vi "SEQ Header Save.vi"(0 "refnum":refnum<file>, 1 "time of 1st frame, \nsec since 1/1/04":dbl format="%.2f", 5 "User Info":string="123456789012345678901234567890123456789", 7 "Description":string="1234567890123456789012345678901234567890123456789012345678901234567890123456789012345678901234567890123456789012345678901234567", 9 "# of Frames":u32=1, 11 "error in":errorcluster, 12 "AOI List":u16[][](array[numeric])) -> (4 "dup refnum":refnum<file>, 15 "error out":errorcluster)   [LabVIEW 2011]
doc: "This VI is used, along with SEQ Body Save, to convert a LabVIEW image array into the SEQ format. SEQ Header Save is run before SEQ Body Save and it records the header information necessary for the SEQ file structure.\n The header information is saved in the following order:\n\"IRN\" - a 3 character string, the first part of any SEQ file.\nUser Info - a 39 character string (or less) for the name of the SEQ's creator.\nDescription - a 127 character string (or less) for a description of the SEQ.\nTime Info - a !!! character string describing the date/time of the SEQ's conception.\nCompression bit - an word integer NOT USED in the LabVIEW format. The original purpose of this int was to differentiate between a compressed SEQ (1) and an uncompressed SEQ (0).\n# of Frames - a word integer of how many frames in the SEQ.\n# of AOIs - a word integers of how many AOIs in the SEQ.\nAOI Table - the AOI table is saved within the header, although in a different format from the AOI file saved in Write SEQ.vi. This table is saved with the four parameters: startx, starty, lengthx, lengthy rather than the AOI List's format of startx, starty, endx, endy.\n\nA note on the bitswapping:\nThe original SEQ file structure stores word integers in a swapped manner to that which LabVIEW produces. This is why it was necessary to swap all word integers.\n\n***This VI was based on the orignal C++ code in v:\\msdev\\convert.cpp."
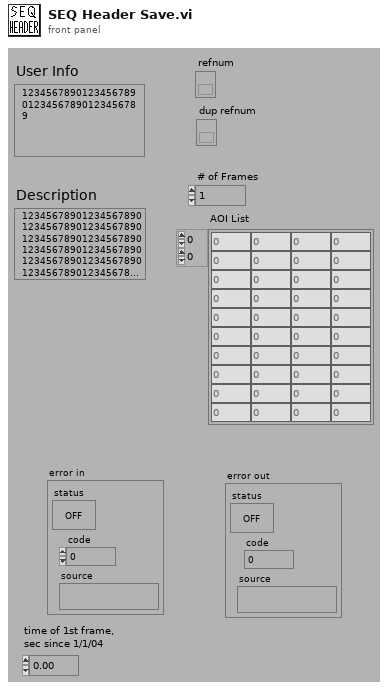
[diagram p1: front panel]
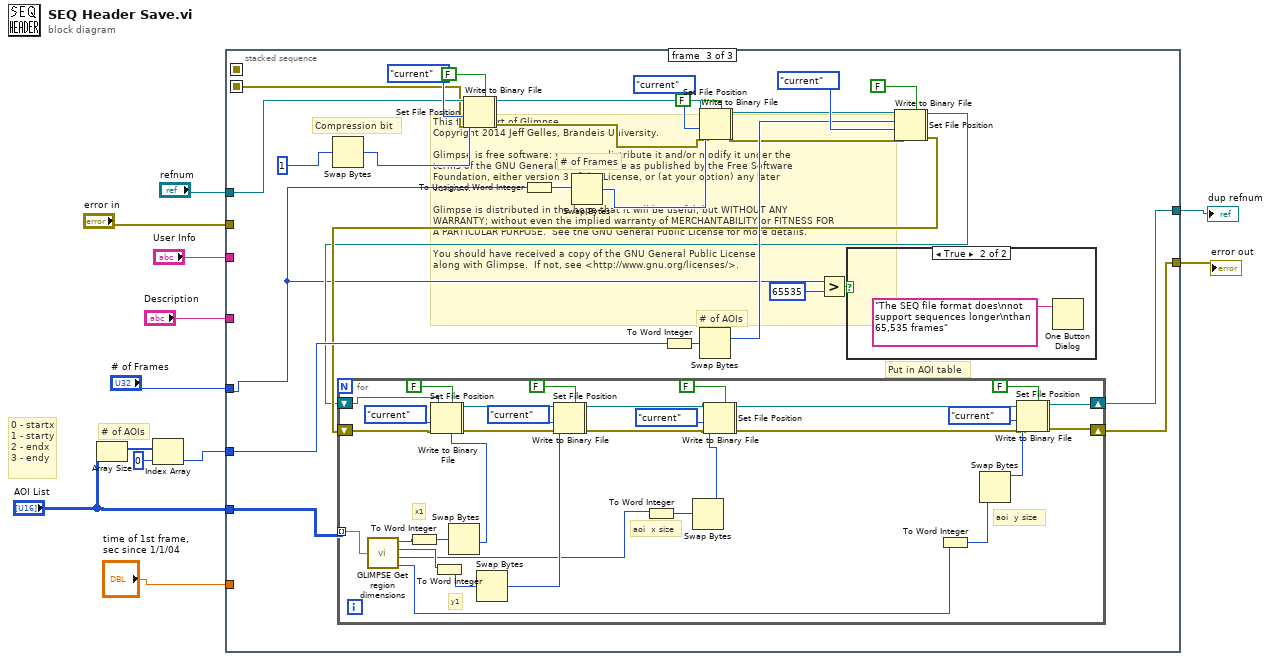
[diagram p0: block diagram]
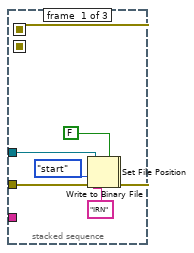
[diagram p2: hidden frame]
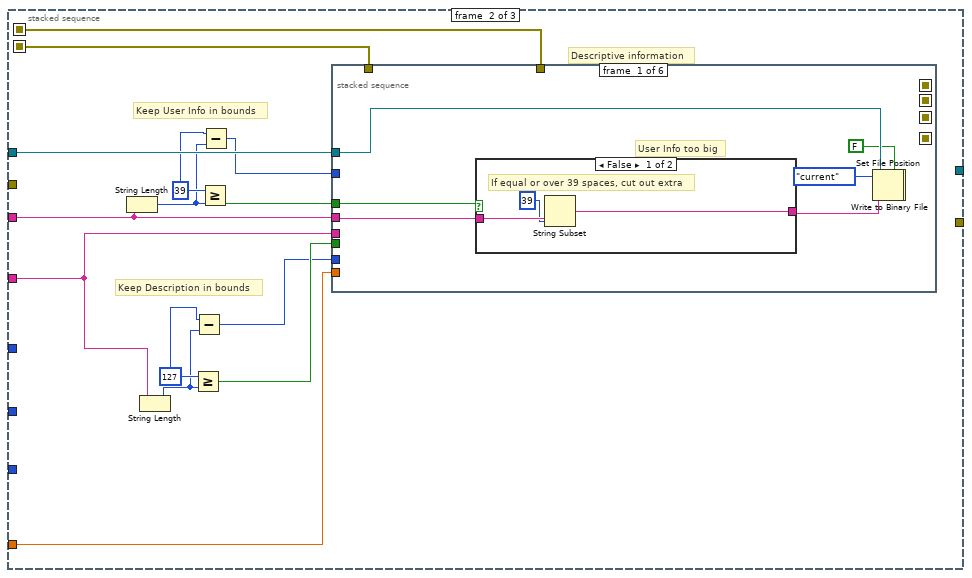
[diagram p3: hidden frame]
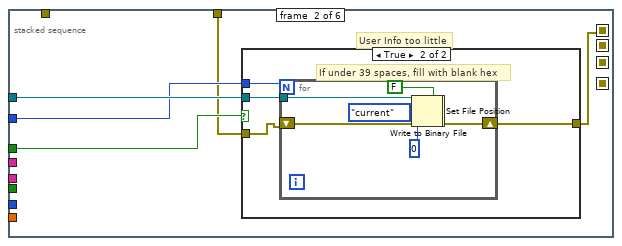
[diagram p5: hidden frame]
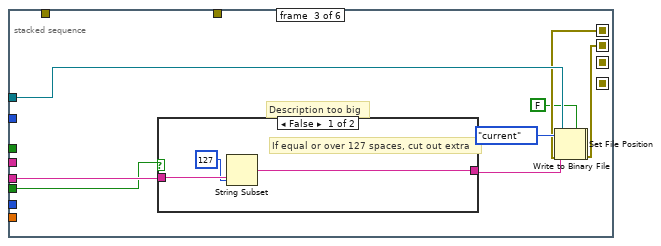
[diagram p7: hidden frame]
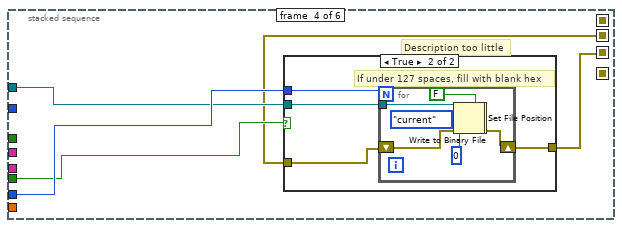
[diagram p9: hidden frame]
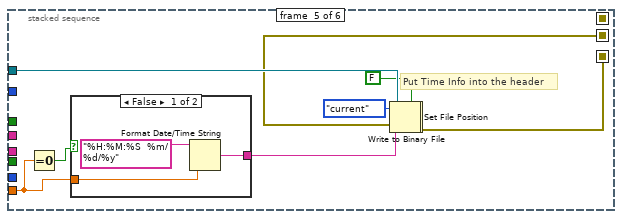
[diagram p11: hidden frame]
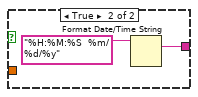
[diagram p12: hidden frame]
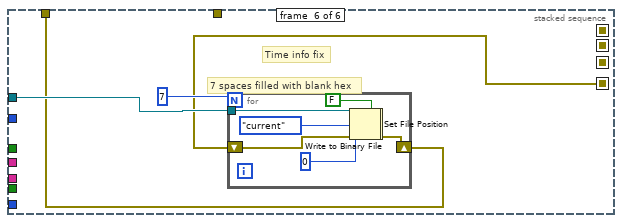
[diagram p13: hidden frame]
diagram:
  # "This file is part of Glimpse. \nCopyright 2014 Jeff Gelles, Brandeis University.    \n\nGlimpse is free software: you can redistribute it and/or modify it under the \nterms of the GNU General Public License as published by the Free Software \nFoundation, either version 3 of the License, or (at your option) any later \nversion.\n\nGlimpse is distributed in the hope that it will be useful, but WITHOUT ANY \nWARRANTY; without even the implied warranty of MERCHANTABILITY or FITNESS FOR \nA PARTICULAR PURPOSE.  See the GNU General Public License for more details.\n\nYou should have received a copy of the GNU General Public License\nalong with Glimpse.  If not, see <http://www.gnu.org/licenses/>."
  # "# of AOIs"
  # "0 - startx\n1 - starty\n2 - endx\n3 - endy"
  n1 = Array Size(array="AOI List") -> (size(s)=w8:i32[])
  n2 = Index Array(array=w8, index=0) -> (element=w6:i32)
  n3 = stacked-sequence {
    seq-local: [w16 _ _] -> [_ w22 _]
    seq-local: [_ w21 _] -> [_ _ w152]
    tunnel: "refnum" -> [w18 w31 w155]
    tunnel: "User Info" -> [_ w24 _]
    tunnel: "Description" -> [_ w26 _]
    tunnel: "# of Frames" -> [_ _ w135]
    tunnel: "AOI List" -> [_ _ w140]
    tunnel: w6 -> [_ _ w143]
    tunnel: "time of 1st frame, \nsec since 1/1/04" -> [_ w23 _]
    tunnel: "error in" -> [w17 _ _]
    tunnel: [_ _ w137] -> w3
    tunnel: [_ _ w136] -> w2
    frame #0 {
      n4 = Set File Position(refnum=w18, from (0:start)=enum16{"start", "end", "current"}."start" ("pos mode (0:2)"), error in=w17) -> (refnum out=w15:refnum<file>, error out=w14:errorcluster)  [unwired: 1 out]
      n5 = Write to Binary File(file (use dialog)=w15, data="IRN", error in=w14, 5:FALSE ("prepend array or string size? (T)")) -> (error out=w16:errorcluster)  [unwired: 4 out]
    }
    frame #1 {
      w30 = 39 ("x")
      w34 = 127 ("x")
      # "Descriptive information"
      # "Keep Description in bounds"
      # "Keep User Info in bounds"
      n6 = String Length(string=w24) -> (length=w29:i32)
      n7 = String Length(string=w26) -> (length=w32:i32)
      n8 = Greater Or Equal?(x=w34, y=w32) -> (x >= y?=w33:bool)
      n9 = Subtract(x=w34, y=w32) -> (x-y=w25:i32)
      n10 = Greater Or Equal?(x=w30, y=w29) -> (x >= y?=w27:bool)
      n11 = Subtract(x=w30, y=w29) -> (x-y=w28:i32)
      n12 = stacked-sequence {
        seq-local: [_ w47 _ _ _ _] -> [_ _ w69 _ _ _]
        seq-local: [_ _ w68 _ _ _] -> [_ _ _ w80 _ _]
        seq-local: [_ _ _ w79 _ _] -> [_ _ _ _ w101 _]
        seq-local: [_ _ _ _ w100 _] -> [_ _ _ _ _ w113]
        tunnel: w24 -> [w39 _ _ _ _ _]
        tunnel: w31 -> [w41 w51 w70 w82 w105 w114]
        tunnel: w28 -> [_ w49 _ _ _ _]
        tunnel: w27 -> [w38 w50 _ _ _ _]
        tunnel: w26 -> [_ _ w72 _ _ _]
        tunnel: w33 -> [_ _ w71 w81 _ _]
        tunnel: w25 -> [_ _ _ w83 _ _]
        tunnel: w23 -> [_ _ _ _ w103 _]
        tunnel: w22 -> [_ w48 _ _ _ _]
        tunnel: [_ _ _ _ _ w112] -> w21
        frame #0 {
          # "User Info too big"
          n13 = case shown="False" w38 {
            tunnel: w39 -> [w45 w46]
            tunnel: [w43 w46] -> w42
            frame False {
              # "If equal or over 39 spaces, cut out extra"
              n14 = String Subset(string=w45, length (rest)=39 ("length")) -> (substring=w43:string)  [unwired: 1 out]
            }
            frame True {
              # "else, nothing"
            }
          }
          n15 = Set File Position(refnum=w41, from (0:start)=enum16{"start", "end", "current"}."current" ("pos mode (0:2)")) -> (refnum out=w37:refnum<file>, error out=w36:errorcluster)  [unwired: 1 in, 1 out]
          n16 = Write to Binary File(file (use dialog)=w37, data=w42, error in=w36, 5:FALSE ("prepend array or string size? (T)")) -> ()  [unwired: 5 out]
        }
        frame #1 {
          # "User Info too little"
          n17 = case shown="True" w50 {
            tunnel: w51 -> [_ w56]
            tunnel: w49 -> [_ w55]
            tunnel: w48 -> [w52 w54]
            tunnel: [w52 w53] -> w47
            frame False {
              # "otherwise, nothing"
            }
            frame True {
              # "If under 39 spaces, fill with blank hex"
              n18 = for {
                N: w55 -> [_]
                tunnel: w56 -> [w63]
                shift-right: [w60] -> w53
                shift-left: w54 -> [w61]
                n19 = Set File Position(refnum=w63, from (0:start)=enum16{"start", "end", "current"}."current" ("pos mode (0:2)"), error in=w61) -> (refnum out=w59:refnum<file>, error out=w58:errorcluster)  [unwired: 1 out]
                n20 = Write to Binary File(file (use dialog)=w59, data=i8 0, error in=w58, 5:FALSE ("prepend array or string size? (T)")) -> (error out=w60:errorcluster)  [unwired: 4 out]
              }
            }
          }
        }
        frame #2 {
          # "Description too big"
          n21 = case shown="False" w71 {
            tunnel: w72 -> [w77 w78]
            tunnel: [w75 w78] -> w74
            frame False {
              # "If equal or over 127 spaces, cut out extra"
              n22 = String Subset(string=w77, length (rest)=127 ("length")) -> (substring=w75:string)  [unwired: 1 out]
            }
            frame True {
              # "else, nothing"
            }
          }
          n23 = Set File Position(refnum=w70, from (0:start)=enum16{"start", "end", "current"}."current" ("pos mode (0:2)"), error in=w69) -> (refnum out=w67:refnum<file>, error out=w66:errorcluster)  [unwired: 1 out]
          n24 = Write to Binary File(file (use dialog)=w67, data=w74, error in=w66, 5:FALSE ("prepend array or string size? (T)")) -> (error out=w68:errorcluster)  [unwired: 4 out]
        }
        frame #3 {
          # "Description too little"
          n25 = case shown="True" w81 {
            tunnel: w82 -> [_ w88]
            tunnel: w83 -> [_ w87]
            tunnel: w80 -> [w84 w86]
            tunnel: [w84 w85] -> w79
            frame False {
              # "else, nothing"
            }
            frame True {
              # "If under 127 spaces, fill with blank hex"
              n26 = for {
                N: w87 -> [_]
                tunnel: w88 -> [w95]
                shift-right: [w92] -> w85
                shift-left: w86 -> [w93]
                n27 = Set File Position(refnum=w95, from (0:start)=enum16{"start", "end", "current"}."current" ("pos mode (0:2)"), error in=w93) -> (refnum out=w91:refnum<file>, error out=w90:errorcluster)  [unwired: 1 out]
                n28 = Write to Binary File(file (use dialog)=w91, data=i8 0, error in=w90, 5:FALSE ("prepend array or string size? (T)")) -> (error out=w92:errorcluster)  [unwired: 4 out]
              }
            }
          }
        }
        frame #4 {
          # "Put Time Info into the header"
          n29 = Equal To 0?(x=w103) -> (x = 0?=w102:bool)
          n30 = case shown="False" w102 {
            tunnel: [w108 w110] -> w104
            tunnel: w103 -> [w107 _]
            frame False {
              n31 = Format Date/Time String(time format string (%c)="%H:%M:%S  %m/%d/%y", seconds (now)=w107) -> (date/time string=w108:string)  [unwired: 1 out]
            }
            frame True {
              n32 = Format Date/Time String(time format string (%c)="%H:%M:%S  %m/%d/%y") -> (date/time string=w110:string)  [unwired: 2 out]
            }
          }
          n33 = Set File Position(refnum=w105, from (0:start)=enum16{"start", "end", "current"}."current" ("pos mode (0:2)"), error in=w101) -> (refnum out=w99:refnum<file>, error out=w98:errorcluster)  [unwired: 1 out]
          n34 = Write to Binary File(file (use dialog)=w99, data=w104, error in=w98, 5:FALSE ("prepend array or string size? (T)")) -> (error out=w100:errorcluster)  [unwired: 4 out]
        }
        frame #5 {
          # "7 spaces filled with blank hex"
          # "Time info fix"
          n35 = for {
            N: 7 -> [_]
            tunnel: w114 -> [w122]
            shift-right: [w119] -> w112
            shift-left: w113 -> [w120]
            n36 = Set File Position(refnum=w122, from (0:start)=enum16{"start", "end", "current"}."current" ("pos mode (0:2)"), error in=w120) -> (refnum out=w118:refnum<file>, error out=w117:errorcluster)  [unwired: 1 out]
            n37 = Write to Binary File(file (use dialog)=w118, data=i8 0, error in=w117, 5:FALSE ("prepend array or string size? (T)")) -> (error out=w119:errorcluster)  [unwired: 4 out]
          }
        }
      }
    }
    frame #2 {
      # "Put in AOI table"
      # "# of AOIs"
      # "# of Frames"
      # "Compression bit"
      n38 = Swap Bytes(anything=u16 1) -> (byte swapped=w154:u16)
      n39 = Set File Position(refnum=w155, from (0:start)=enum16{"start", "end", "current"}."current" ("pos mode (0:2)"), error in=w152) -> (refnum out=w126:refnum<file>, error out=w125:errorcluster)  [unwired: 1 out]
      n40 = Write to Binary File(file (use dialog)=w126, data=w154, error in=w125, 5:FALSE ("prepend array or string size? (T)")) -> (refnum out=w148:refnum<file>, error out=w147:errorcluster)  [unwired: 3 out]
      n41 = To Unsigned Word Integer(number=w135) -> (unsigned 16bit integer=w150:u16)
      n42 = Swap Bytes(anything=w150) -> (byte swapped=w149:u16)
      n43 = To Word Integer(number=w143) -> (16bit integer=w144:i16)
      n44 = Set File Position(refnum=w148, from (0:start)=enum16{"start", "end", "current"}."current" ("pos mode (0:2)"), error in=w147) -> (refnum out=w129:refnum<file>, error out=w128:errorcluster)  [unwired: 1 out]
      n45 = Swap Bytes(anything=w144) -> (byte swapped=w145:i16)
      n46 = Write to Binary File(file (use dialog)=w129, data=w149, error in=w128, 5:FALSE ("prepend array or string size? (T)")) -> (refnum out=w141:refnum<file>, error out=w142:errorcluster)  [unwired: 3 out]
      n47 = Greater?(x=w135, y=u32 65535) -> (0:w133:bool)
      n48 = case shown="True" w133 {
        frame False {
        }
        frame True {
          n49 = One Button Dialog(message="The SEQ file format does\nnot support sequences longer\nthan 65,535 frames") -> ()  [unwired: 2 out]
        }
      }
      n50 = Set File Position(refnum=w141, from (0:start)=enum16{"start", "end", "current"}."current" ("pos mode (0:2)"), error in=w142) -> (refnum out=w132:refnum<file>, error out=w131:errorcluster)  [unwired: 1 out]
      n51 = Write to Binary File(file (use dialog)=w132, data=w145, error in=w131, 5:FALSE ("prepend array or string size? (T)")) -> (refnum out=w138:refnum<file>, error out=w139:errorcluster)  [unwired: 3 out]
      n52 = for {
        tunnel: w140 -> [w186] mode=indexing
        shift-right: [w170] -> w137
        shift-left: w138 -> [w193]
        shift-right: [w171] -> w136
        shift-left: w139 -> [w192]
        # "aoi  y size"
        # "aoi  x size"
        # "y1"
        # "x1"
        n53 = call "GLIMPSE Get region dimensions.vi"("x1y1x2y2"=w186) -> ("y size"=w177:u16, "x size"=w176:u16, "y origin"=w184:u16, "x origin"=w185:u16)  [unwired: 7 out]
        n54 = To Word Integer(number=w185) -> (16bit integer=w196:i16)
        n55 = Set File Position(refnum=w193, from (0:start)=enum16{"start", "end", "current"}."current" ("pos mode (0:2)"), error in=w192) -> (refnum out=w160:refnum<file>, error out=w159:errorcluster)  [unwired: 1 out]
        n56 = To Word Integer(number=w184) -> (16bit integer=w191:i16)
        n57 = Swap Bytes(anything=w196) -> (byte swapped=w195:i16)
        n58 = Write to Binary File(file (use dialog)=w160, data=w195, error in=w159, 5:FALSE ("prepend array or string size? (T)")) -> (refnum out=w188:refnum<file>, error out=w189:errorcluster)  [unwired: 3 out]
        n59 = Swap Bytes(anything=w191) -> (byte swapped=w187:i16)
        n60 = Set File Position(refnum=w188, from (0:start)=enum16{"start", "end", "current"}."current" ("pos mode (0:2)"), error in=w189) -> (refnum out=w163:refnum<file>, error out=w162:errorcluster)  [unwired: 1 out]
        n61 = Write to Binary File(file (use dialog)=w163, data=w187, error in=w162, 5:FALSE ("prepend array or string size? (T)")) -> (refnum out=w174:refnum<file>, error out=w175:errorcluster)  [unwired: 3 out]
        n62 = To Word Integer(number=w176) -> (16bit integer=w183:i16)
        n63 = Swap Bytes(anything=w183) -> (byte swapped=w182:i16)
        n64 = Set File Position(refnum=w174, from (0:start)=enum16{"start", "end", "current"}."current" ("pos mode (0:2)"), error in=w175) -> (refnum out=w166:refnum<file>, error out=w165:errorcluster)  [unwired: 1 out]
        n65 = Write to Binary File(file (use dialog)=w166, data=w182, error in=w165, 5:FALSE ("prepend array or string size? (T)")) -> (refnum out=w173:refnum<file>, error out=w172:errorcluster)  [unwired: 3 out]
        n66 = To Word Integer(number=w177) -> (16bit integer=w178:i16)
        n67 = Swap Bytes(anything=w178) -> (byte swapped=w179:i16)
        n68 = Set File Position(refnum=w173, from (0:start)=enum16{"start", "end", "current"}."current" ("pos mode (0:2)"), error in=w172) -> (refnum out=w169:refnum<file>, error out=w168:errorcluster)  [unwired: 1 out]
        n69 = Write to Binary File(file (use dialog)=w169, data=w179, error in=w168, 5:FALSE ("prepend array or string size? (T)")) -> (refnum out=w170:refnum<file>, error out=w171:errorcluster)  [unwired: 3 out]
      }
    }
  }
  "error out" <- w2
  "dup refnum" <- w3
